vi "trash_Write Local Manager Address.vi"(8 "error in (no error)":errorcluster, 10 "Local Manager Address":string, 11 "CIFCorePlugin in":refnum<class "CIFCorePlugin.lvclass">) -> (0 "error out":errorcluster, 3 "CIFCorePlugin out":refnum<class "CIFCorePlugin.lvclass">)   [LabVIEW 2021]
uses:
  CIFCorePlugin.lvclass/CIFCorePlugin.ctl
  CIFCorePlugin.lvclass
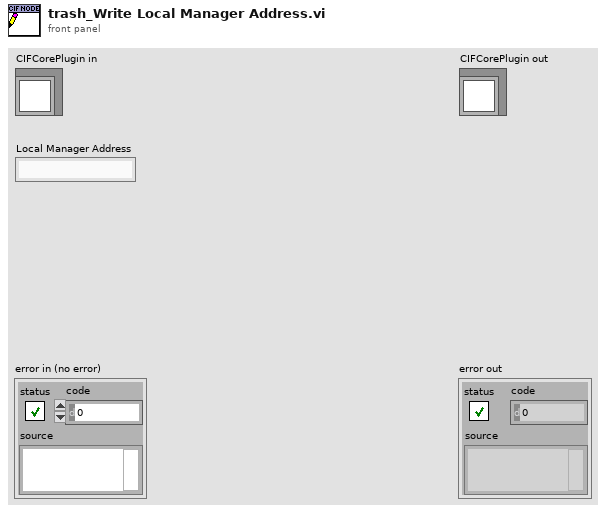
[diagram p1: front panel]
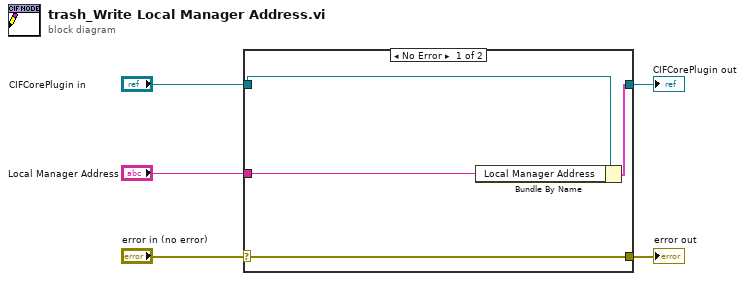
[diagram p0: block diagram]
diagram:
  n1 = case shown="No Error" "error in (no error)" {
    selector: "error in (no error)" -> [w9 w10]
    tunnel: [w9 w10] -> w4
    tunnel: [w7 w11] -> w2
    tunnel: "CIFCorePlugin in" -> [w8 w11]
    tunnel: "Local Manager Address" -> [w6 _]
    frame No Error {
      n2 = Bundle By Name(cluster=w8, "Local Manager Address"=w6) -> (w7:cluster{})
    }
    frame Error {
    }
  }
  "error out" <- w4
  "CIFCorePlugin out" <- w2
